vi "Construct Error Cluster.vi"(1 "Error In":errorcluster, 2 "Reason":string, 3 "Call Chain":bool=TRUE, 4 "Error Code":i32=8000) -> (0 "Error Out":errorcluster)   [LabVIEW 2018]
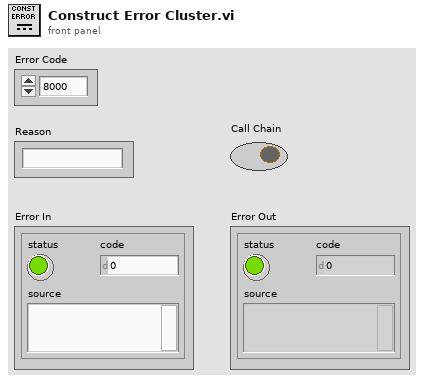
[diagram p1: front panel]
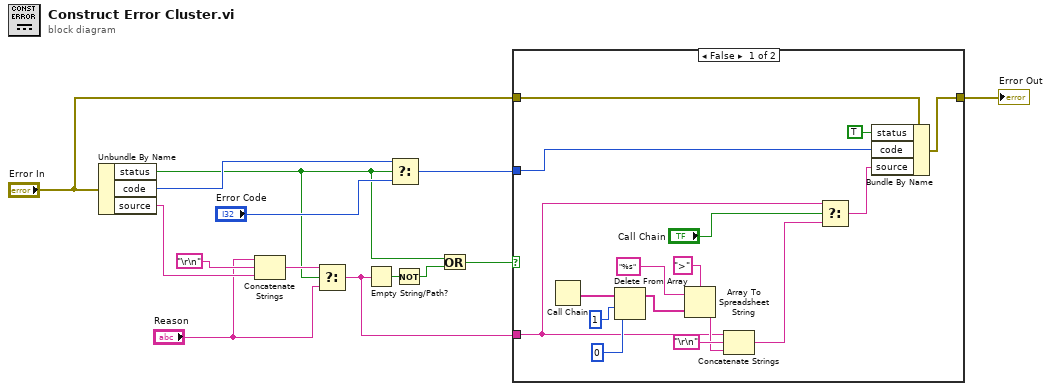
[diagram p0: block diagram]
diagram:
  n1 = Unbundle By Name("Error In") -> ("status"=w1:bool, "code"=w9:i32, "source"=w11:string)
  n2 = Concatenate Strings("Reason", "\r\n", w11) -> (w14:string)
  n3 = Select(t=w14, s=w1, f="Reason") -> (s? t:f=w3:string)
  n4 = Empty String/Path?(string/path=w3) -> (empty?=w13:bool)
  n5 = Select(t=w9, s=w1, f="Error Code") -> (s? t:f=w6:i32)
  n6 = Not(x=w13) -> (.not. x?=w12:bool)
  n7 = Or(x=w1, y=w12) -> (x .or. y?=w7:bool)
  n8 = case shown="False" w7 {
    tunnel: w6 -> [w18 _]
    tunnel: "Error In" -> [w24 w31]
    tunnel: w3 -> [w21 _]
    tunnel: [w23 w31] -> w2
    frame False {
      n9 = Call Chain() -> (call chain=w29:string[])
      n10 = Delete From Array(array=w29, length=1, index=0) -> (array with subset deleted=w26:string[])  [unwired: 1 out]
      n11 = Array To Spreadsheet String(delimiter (Tab)=">", array=w26, 3:"%s" ("format string")) -> (spreadsheet string=w25:string)
      n12 = Concatenate Strings(w21, "\r\n", w25) -> (w22:string)
      n13 = Select(t=w21, s="Call Chain", f=w22) -> (s? t:f=w19:string)
      n14 = Bundle By Name(cluster=w24, "status"=TRUE, "code"=w18, "source"=w19) -> (w23:errorcluster)
    }
    frame True {
      # "Empty string means no error"
    }
  }
  "Error Out" <- w2
